vi "DFD 2-Band Filter Bank Reconstruction (Wfm).vi"(7 "init? (F)":bool, 8 "error in (no error)":errorcluster, 9 "filter bank in":T1 {"mFBank_SynthesisFilters"."mMRate_SumWl" min=1 max=32 step=1; "mFBank_SynthesisFilters"."mMRate_InputIwl" min=1 max=32 step=1; "mFBank_SynthesisFilters"."mMRate_GainWl" min=1 max=32 step=1; "mFBank_SynthesisFilters"."mMRate_OutputWl" min=1 max=32 step=1; "mFBank_SynthesisFilters"."mMRate_InputWl" min=1 max=32 step=1; "mFBank_SynthesisFilters"."mMRate_CoefWl" min=1 max=32 step=1; "mFBank_SynthesisFilters"."mMRate_Mode" items=["Default"=-1, "No Rate Change"=0, "Interpolation"=1, "Decimation"=2, "Interpolated"=3, "Rational"=4]; "mFBank_AnalysisFilters"."mMRate_SumWl" min=1 max=32 step=1; "mFBank_AnalysisFilters"."mMRate_InputIwl" min=1 max=32 step=1; "mFBank_AnalysisFilters"."mMRate_GainWl" min=1 max=32 step=1; "mFBank_AnalysisFilters"."mMRate_OutputWl" min=1 max=32 step=1; "mFBank_AnalysisFilters"."mMRate_InputWl" min=1 max=32 step=1; "mFBank_AnalysisFilters"."mMRate_CoefWl" min=1 max=32 step=1; "mFBank_AnalysisFilters"."mMRate_Mode" items=["Default"=-1, "No Rate Change"=0, "Interpolation"=1, "Decimation"=2, "Interpolated"=3, "Rational"=4]; "mFBank_Type" items=["Uniform", "Non-Uniform"]}, 10 "highpass band":waveform(dbl)={"t0"=timestamp(0 s since 1904-01-01), "dt"=0.0, "Y"=[]}, 11 "lowpass band":waveform(dbl)={"t0"=timestamp(0 s since 1904-01-01), "dt"=0.0, "Y"=[]}) -> (0 "error out":errorcluster, 3 "signal out":waveform(dbl))   [LabVIEW 2017, in "NI_DigFilter_FilterBank.lvlib"]
doc: "Reconstructs a signal from a lowpass band signal and a highpass band signal continuously with a 2-band filter bank."
uses:
  <vilib>/addons/Digital Filter Design/NI_DigFilter_FilterBank.lvlib
  <vilib>/addons/Digital Filter Design/FilterBank.llb/Object/DFD Filter Bank Obj.ctl
  <vilib>/addons/Digital Filter Design/_Objects.llb/DFD Multirate Filter Obj.ctl
  <vilib>/addons/Digital Filter Design/_Objects.llb/DFD Multirate Mode.ctl
  <vilib>/addons/Digital Filter Design/_Objects.llb/DFD Coef Norm Type.ctl
  <vilib>/addons/Digital Filter Design/_Objects.llb/DFD Round-off Mode.ctl
  <vilib>/addons/Digital Filter Design/_Objects.llb/DFD FXP MRate Multiply Mode.ctl
  <vilib>/addons/Digital Filter Design/FilterBank.llb/Object/DFD Filter Bank Processing Method.ctl
  <vilib>/addons/Digital Filter Design/FilterBank.llb/Object/DFD Filter Bank Type.ctl
  <vilib>/addons/Digital Filter Design/FilterBank.llb/Process/DFD 2-Band Filter Bank Reconstruction with State (Wfm).vi
  <vilib>/addons/Digital Filter Design/NI_DigFilter_Process.lvlib
  <vilib>/addons/Digital Filter Design/NI_DigFilterLicensed.lvlib
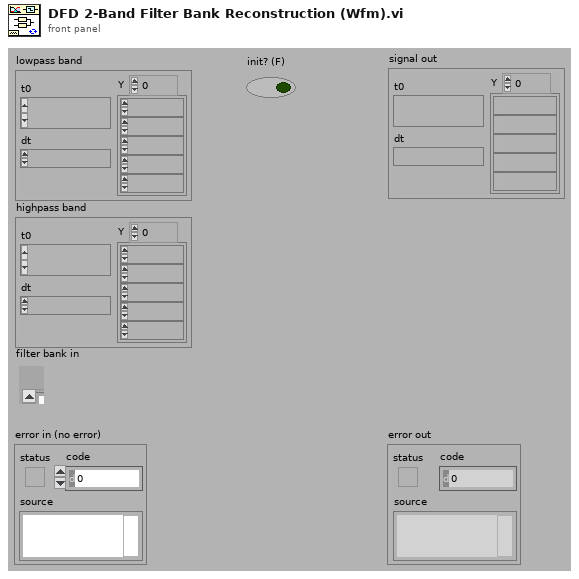
[diagram p1: front panel]
types:
  T1 = typedef "NI_DigFilter_FilterBank.lvlib/DFD Filter Bank Obj.ctl" = cluster{"mFBank_AnalysisFilters":T2[], "mFBank_SynthesisFilters":T2[], "mFBank_#Bands":i32, "mFBank_ProcMethod":T7, "mFBank_Coeffs":dbl[], "mFBank_Gain":dbl, "mFBank_Delay":i32, "mFBank_Type":T8}
  T2 = typedef "NI_DigFilterLicensed.lvlib/DFD Multirate Filter Obj.ctl" = cluster{"mMRate_Structure":enum16{"CIC", "FIR", "IIR", "Lattice"}, "mMRate_Mode":T3, "mMRate_Factor":i32, "mMRate_FIRParams":cluster{"mMRate_FIR_H":dbl[], "mMRate_FIR_IsNyquist?":bool, "mMRate_FIR_IsSymmetric?":bool}, "mMRate_CICParams":cluster{"mMRate_CIC_#Stage":i32, "mMRate_CIC_Lag":i32, "mMRate_CIC_Type":enum16{"Lowpass", "Highpass"}}, "mMRate_Order":i32, "mMRate_Version":string, "mMRate_Comments":string, "mMRate_RationalFactor":cluster{"mMRate_L":i32, "mMRate_M":i32}, "mMRate_Fs":dbl, "mMRate_Quantized?":bool, "mMRate_QFilterGain":dbl, "mMRate_CoefWl":i16, "mMRate_Scaling":cluster{"mMRate_ScaleByPowerOf2?":bool, "mMRate_ScaleType":T4}, "mMRate_InputWl":i16, "mMRate_OutputWl":i16, "mMRate_OutputMode":T5, "mMRate_MultMode":T6, "mMRate_BitPruning":bool, "mMRate_GainWl":i16, "mMRate_OutputFwl":i16, "mMRate_SumIwl":i16, "mMRate_InputIwl ":i16, "mMRate_SumWl":i16, "mMRate_CoefIwl":i16}
  T3 = typedef "NI_DigFilterLicensed.lvlib/DFD Multirate Mode.ctl" = i16
  T4 = typedef "NI_DigFilterLicensed.lvlib/DFD Coef Norm Type.ctl" = enum16{"No Norm", "Time Domain 1-Norm", "Time Domain 2-Norm", "Time Domain Inf-Norm"}
  T5 = typedef "NI_DigFilterLicensed.lvlib/DFD Round-off Mode.ctl" = enum16{"Nearest", "Truncation"}
  T6 = typedef "NI_DigFilterLicensed.lvlib/DFD FXP MRate Multiply Mode.ctl" = enum16{"Truncated", "Full"}
  T7 = typedef "NI_DigFilter_FilterBank.lvlib/DFD Filter Bank Processing Method.ctl" = enum16{"General", "2-Band QMF Lattice", "Cosine-Modulated"}
  T8 = typedef "NI_DigFilter_FilterBank.lvlib/DFD Filter Bank Type.ctl" = u16
  T9 = typedef "NI_DigFilter_FilterBank.lvlib/DFD Bank Obj.ctl" = cluster{"mBank_Filters":T2[], " mBank_#Bands":i32, "mBank_ProcMethod":T7, "mBank_Coeffs":dbl[], "mBank_Gain":dbl, "mBank_Type":T8}
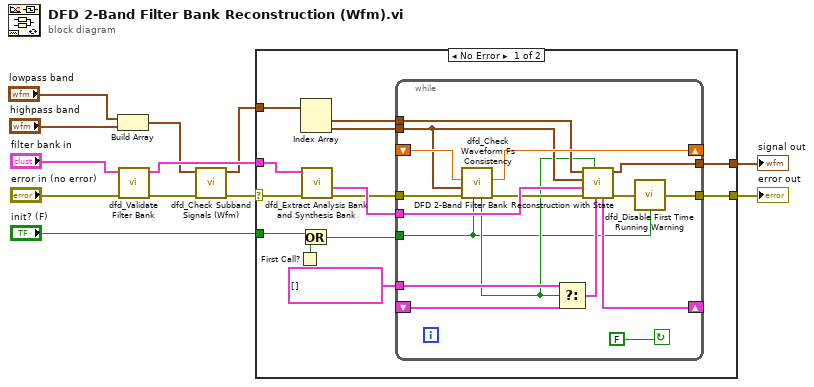
[diagram p0: block diagram]
diagram:
  n1 = Build Array("lowpass band", "highpass band") -> (w5:waveform(dbl)[])
  n2 = call <vilib>:"dfd_Validate Filter Bank.vi"("error in (no error)"="error in (no error)", "filter banks in"="filter bank in") -> ("error out"=w4:errorcluster, "filter bank out"=w8:T1)  [unwired: 7 in, 1 out]
  n3 = call <vilib>:"dfd_Check Subband Signals (Wfm).vi"("error in (no error)"=w4, "subband signals"=w5) -> ("error out"=w3:errorcluster, "dup subband signals"=w2:waveform(dbl)[])  [unwired: 8 in]
  n4 = case shown="No Error" w3 {
    selector: w3 -> [w21 w43]
    tunnel: w8 -> [w23 _]
    tunnel: [w24 w43] -> w12
    tunnel: [w25 _] -> w11
    tunnel: "init? (F)" -> [w17 _]
    tunnel: w2 -> [w15 _]
    frame No Error {
      n5 = First Call?() -> (First Call?: T/F=w19:bool)
      n6 = Index Array(array=w15) -> (element #1=w14:waveform(dbl), element #2=w13:waveform(dbl))  [unwired: 2 in]
      n7 = Or(x=w17, y=w19) -> (x .or. y?=w18:bool)
      n8 = call <vilib>:"dfd_Extract Analysis Bank and Synthesis Bank.vi"("error in (no error)"=w21, "filter banks in"=w23) -> ("error out"=w20:errorcluster, "synthesis bank"=w22:T9)  [unwired: 6 in, 2 out]
      n9 = while {
        shift-right: [w34] -> _
        shift-left: _ -> [w35]
        tunnel: cluster{dbl[]}[] [] -> [w42]
        shift-right: [w38] -> _
        shift-left: _ -> [w41]
        tunnel: w18 -> [w26]
        tunnel: w20 -> [w32]
        tunnel: [w37] -> w25
        tunnel: [w28] -> w24
        tunnel: w22 -> [w36]
        tunnel: w14 -> [w31]
        tunnel: w13 -> [w30]
        stop <- FALSE continue-if-true
        n10 = call <vilib>:"dfd_Check Waveform Fs Consistency.vi"("init in"=w26, "error in (no error)"=w32, "signal in"=w30, "dt in"=w35) -> ("error out"=w33:errorcluster, "dt out"=w34:dbl, "init out"=w27:bool)  [unwired: 5 out]
        n11 = Select(t=w42, s=w27, f=w41) -> (s? t:f=w39:cluster{"state ":dbl[]}[])
        n12 = call-poly <vilib>:"DFD 2-Band Filter Bank Reconstruction with State.vi"("state in"=w39, "init? (F)"=w27, "error in (no error)"=w33, "synthesis bank"=w36, "highpass band"=w30, "lowpass band"=w31) -> ("error out"=w29:errorcluster, "y"=w37:waveform(dbl), "state out"=w38:cluster{"state ":dbl[]}[])  [unwired: 3 in]
        n13 = call <vilib>:"dfd_Disable First Time Running Warning.vi"("error in"=w29, "disable?"=w26) -> ("error out"=w28:errorcluster)
      }
    }
    frame Error {
    }
  }
  "signal out" <- w11
  "error out" <- w12
